vi "MySetRateANdField (SubVI).vi"(8 "error in (no error)":errorcluster, 9 "Target B (T)":dbl, 10 "Sweep rate":dbl, 11 "VISA Refnum in":refnum<visa-resource-name>) -> (0 "error out":errorcluster, 3 "VISA Refnum out":refnum<visa-resource-name>)   [LabVIEW 2025, in "MyTriton.lvlib"]
uses:
  MyTriton.lvlib
panel:
  in  "READ Response?":bool
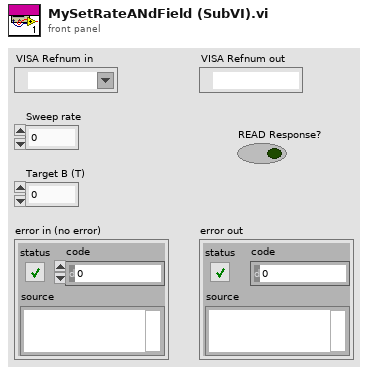
[diagram p1: front panel]
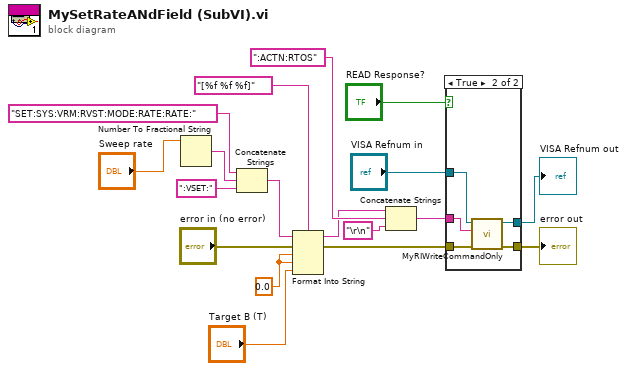
[diagram p0: block diagram]
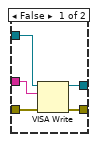
[diagram p2: hidden frame]
diagram:
  w17 = 0.0
  n1 = Number To Fractional String(number="Sweep rate") -> (F-format string=w15:string)  [unwired: 3 in]
  n2 = Concatenate Strings("SET:SYS:VRM:RVST:MODE:RATE:RATE:", w15, ":VSET:") -> (w16:string)
  n3 = Format Into String(format string="[%f %f %f]", initial string=w16, error in="error in (no error)", w17, w17, "Target B (T)") -> (resulting string=w10:string, error out=w4:errorcluster)
  n4 = Concatenate Strings(w10, ":ACTN:RTOS", "\r\n" ("string")) -> (w5:string)
  n5 = case shown="True" "READ Response?" {
    tunnel: "VISA Refnum in" -> [w22 w28]
    tunnel: w5 -> [w21 w27]
    tunnel: w4 -> [w23 w26]
    tunnel: [w20 w25] -> w3
    tunnel: [w19 w24] -> w2
    frame False {
      n6 = VISA Write(VISA resource name=w22, write buffer=w21, error in (no error)=w23) -> (VISA resource name out=w20:refnum<visa-resource-name>, error out=w19:errorcluster)  [unwired: 1 out]
    }
    frame True {
      n7 = call "MyRIWriteCommandOnly.vi"("error in (no error)"=w26, "Command"=w27, "VISA resource name in"=w28) -> ("error out"=w24:errorcluster, "VISA resource name out"=w25:refnum<visa-resource-name>)  [unwired: 7 in]
    }
  }
  "VISA Refnum out" <- w3
  "error out" <- w2
